vi "ReadWrite CSV.vi"(6 "Task":enum16{"Save", "Read"}(ring)=enum."Read", 11 "csv?":bool) -> (3 "csv Out":bool)   [LabVIEW 2022 SP3]
panel:
  out "Pref Path":path
  out "text":string
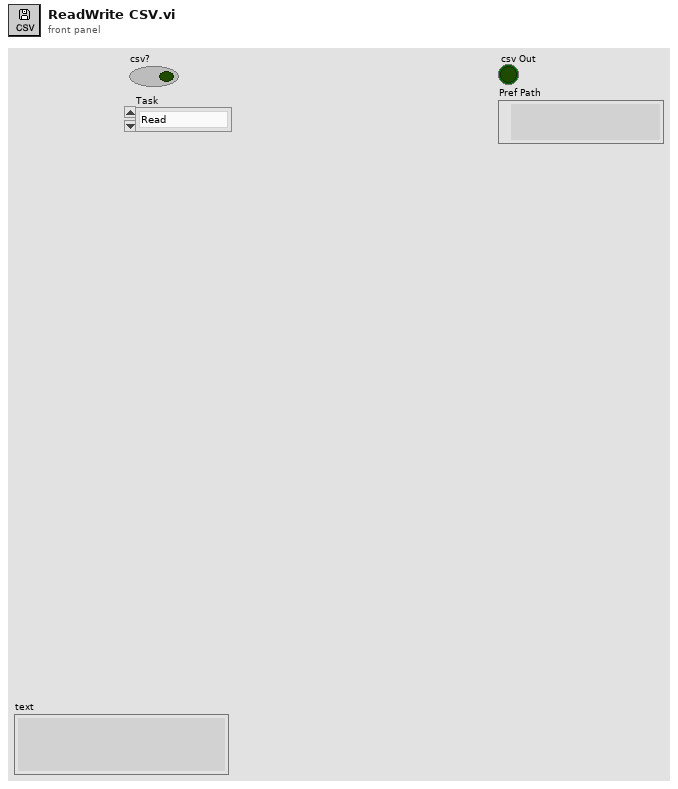
[diagram p1: front panel]
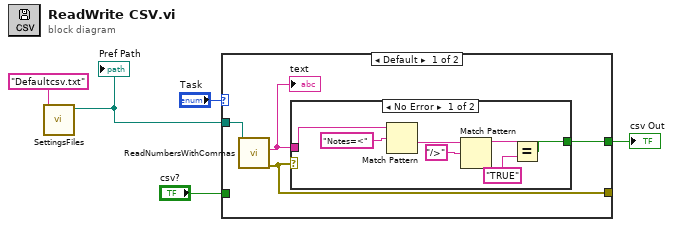
[diagram p0: block diagram]
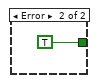
[diagram p2: hidden frame]
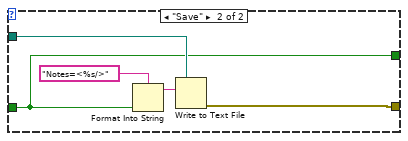
[diagram p3: hidden frame]
diagram:
  n1 = call "SettingsFiles.vi"("settings file name"="Defaultcsv.txt" ("name or relative path")) -> ("file path"=w2:path)  [unwired: 9 in, 1 out]
  "Pref Path" <- w2
  n2 = case shown="Default" "Task" {
    tunnel: "csv?" -> [_ w18]
    tunnel: w2 -> [w8 w22]
    tunnel: [w6 w19] -> _
    tunnel: [w9 w18] -> w5
    frame Default {
      n3 = call "ReadNumbersWithCommas.vi"("file (use dialog)"=w8) -> ("error out"=w6:errorcluster, "text"=w7:string)  [unwired: 7 in, 2 out]
      "text" <- w7
      n4 = case shown="No Error" w6 {
        tunnel: [w11 TRUE] -> w9
        tunnel: w7 -> [w16 _]
        frame No Error {
          n5 = Match Pattern(string=w16, regular expression="Notes=<" ("format string")) -> (after substring=w15:string)  [unwired: 1 in, 3 out]
          n6 = Match Pattern(string=w15, regular expression="/>" ("format string")) -> (before substring=w12:string)  [unwired: 1 in, 3 out]
          n7 = Equal?(x=w12, y="TRUE" ("format string")) -> (x = y?=w11:bool)
        }
        frame Error {
        }
      }
    }
    frame "Save" {
      n8 = Format Into String(format string="Notes=<%s/>", w18) -> (resulting string=w21:string)  [unwired: 2 in, 1 out]
      n9 = Write to Text File(file (use dialog)=w22, text=w21) -> (error out=w19:errorcluster)  [unwired: 2 in, 2 out]
    }
  }
  "csv Out" <- w5
